vi "Get Request.vi"(8 "error in (no error)":errorcluster, 10 "timeout in ms (-1)":i32=-1, 11 "output in":refnum<class "Output.lvclass">) -> (0 "error out":errorcluster, 1 "timed out?":bool, 2 "request.lvclass":refnum<class "request.lvclass">, 3 "output out":refnum<class "Output.lvclass">)   [LabVIEW 2015, in "Output.lvclass"]
uses:
  Output.lvclass
  request/request.lvclass
  Output.lvclass/Output.ctl
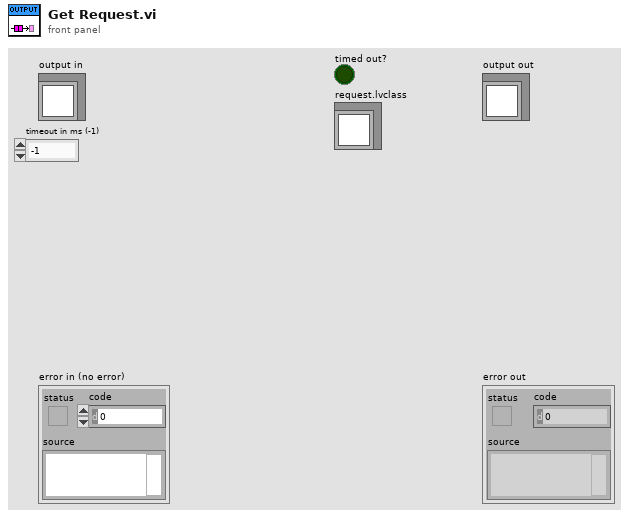
[diagram p1: front panel]
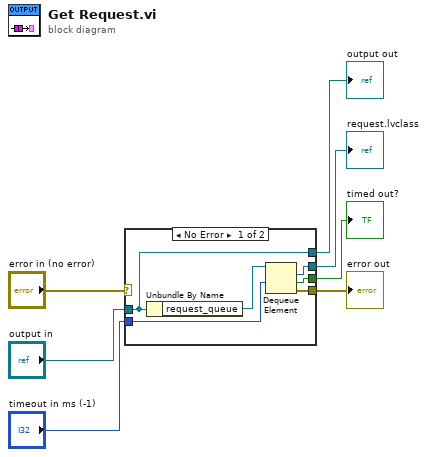
[diagram p0: block diagram]
diagram:
  n1 = case shown="No Error" "error in (no error)" {
    selector: "error in (no error)" -> [_ w15]
    tunnel: [w11 w15] -> w6
    tunnel: [w13 w14] -> w4
    tunnel: "output in" -> [w13 w14]
    tunnel: "timeout in ms (-1)" -> [w10 _]
    tunnel: [w9 _] -> w2
    tunnel: [w8 _] -> w1
    frame No Error {
      n2 = Unbundle By Name(w13) -> ("request_queue"=w12:refnum<queue>)
      n3 = Dequeue Element(queue=w12, timeout in ms (-1)=w10) -> (element=w8:refnum<class "request.lvclass">, timed out?=w9:bool, error out=w11:errorcluster)  [unwired: 1 in, 1 out]
    }
    frame Error {
    }
  }
  "error out" <- w6
  "output out" <- w4
  "timed out?" <- w2
  "request.lvclass" <- w1
